vi "Starter Kit 2.0 Roaming - Kinect.vi"() -> ()   [LabVIEW 2010]
doc: "This VI demonstrates how to control the Robotics Starter Kit 2.0 robot. It is deployed to an sbRIO-9632, then run on the Real-Time controller."
uses:
  <vilib>/Utility/AngleManip/NI_AngleManipulation.lvlib
  <vilib>/Utility/AngleManip/Degrees to Radians (Scalar DBL).vi
  <vilib>/Platform/TimedLoop/XDataNode/XDataNode.xnode
  <vilib>/Platform/TimedLoop/XDataNode/timing_clust.ctl
  <vilib>/Platform/TimedLoop/XDataNode/XDNodeRunTimeDep.lvlib
  <vilib>/Platform/TimedLoop/XDataNode/wakeup.ctl
  <vilib>/Platform/TimedLoop/XDataNode/nitl_modes.ctl
  <vilib>/robotics/Steering/Steering Frame/NI_Robotics_Steering Frame.lvclass
  <vilib>/robotics/Steering/Steering Frame/Apply Steering Frame Velocity to Motors.vi
  <vilib>/robotics/Starter Kit/Host Interface/NI_Robotics_Starter Kit Host.lvclass
  <vilib>/robotics/Utilities/Scan Angles/NI_Robotics_Scan Angles.lvlib
  <vilib>/robotics/Starter Kit/2.0/NI_Robotics_Starter Kit Host_2.0.lvlib
  <vilib>/robotics/Starter Kit/2.0/9632 Host Interface/NI_Robotics_Starter Kit Host_9632_2.0.lvclass
  <vilib>/robotics/Obstacle Avoidance/Simple Vector Field Histogram/Gap Description.ctl
  <vilib>/robotics/Obstacle Avoidance/Simple Vector Field Histogram/NI_Robotics_Simple Vector Field Histogram.lvlib
  <vilib>/robotics/Obstacle Avoidance/Simple Vector Field Histogram/Obstacle Description.ctl
  Kinect VIs/Kinect Heading Data.ctl
panel:
  out "Sensor Data":cluster{"angles (deg)":dbl[], "distances":dbl[]}(graph)
  in  "stop":bool
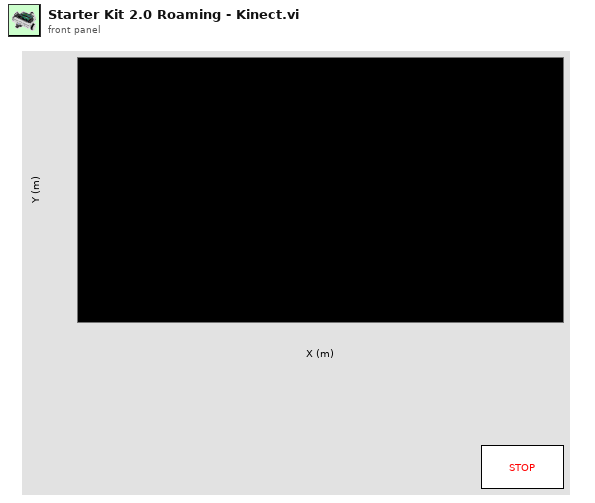
[diagram p1: front panel]
types:
  T1 = typedef "Kinect Heading Data.ctl" = cluster{"largest gap":T2, "nearest obstacle":T3, "obstacle within panic range":bool}
  T2 = typedef "NI_Robotics_Simple Vector Field Histogram.lvlib/Gap Description.ctl" = cluster{"angle to gap":dbl, "size of gap":dbl}
  T3 = typedef "NI_Robotics_Simple Vector Field Histogram.lvlib/Obstacle Description.ctl" = cluster{"angle to obstacle":dbl, "distance to obstacle":dbl}
  T4 = typedef "XDNodeRunTimeDep.lvlib/timing_clust.ctl" = cluster{"Expected End [f-1]":u64, "Actual End [f-1]":u64, "Finished Late? [f-1]":bool, "Expected End [i-1]":u64, "Actual End [i-1]":u64, "Finished Late? [i-1]":bool, "Expected Start [i]":u64, "Actual Start [i]":u64, "Expected Start [f]":u64, "Actual Start [f]":u64, "Source Name":string, "Structure Name":string, "Period":i64, "Deadline":i64, "Offset":i64, "Start":i64, "Priority":i32, "Timeout":i32, "Mode":T5, "Wakeup Reason":T6, "Error":errorcluster, "Source Type":string, "Secondary Source Type":string, "Global End Time":u64, "Global Start Time":u64, "Frame Duration":u64, "Iteration Duration":u64, "Assigned CPU":i32, "I/O Scan Engine Mode":u32}
  T5 = typedef "XDNodeRunTimeDep.lvlib/nitl_modes.ctl" = enum32{"No Change", "Process missed periods, maintain original phase", "Discard missed periods, maintain original phase", "Process missed periods, ignore original phase", "Discard missed periods, ignore original phase"}
  T6 = typedef "XDNodeRunTimeDep.lvlib/wakeup.ctl" = enum32{"Normal", "Aborted", "Asynchronous wakeup", "Timing source error", "Timed loop error", "Timeout"}
  T7 = typedef "NI_Robotics_Scan Angles.lvlib/Scan Angle Data.ctl" = cluster{"angles":dbl[], "distances":dbl[], "current index":i32, "previous index":i32}
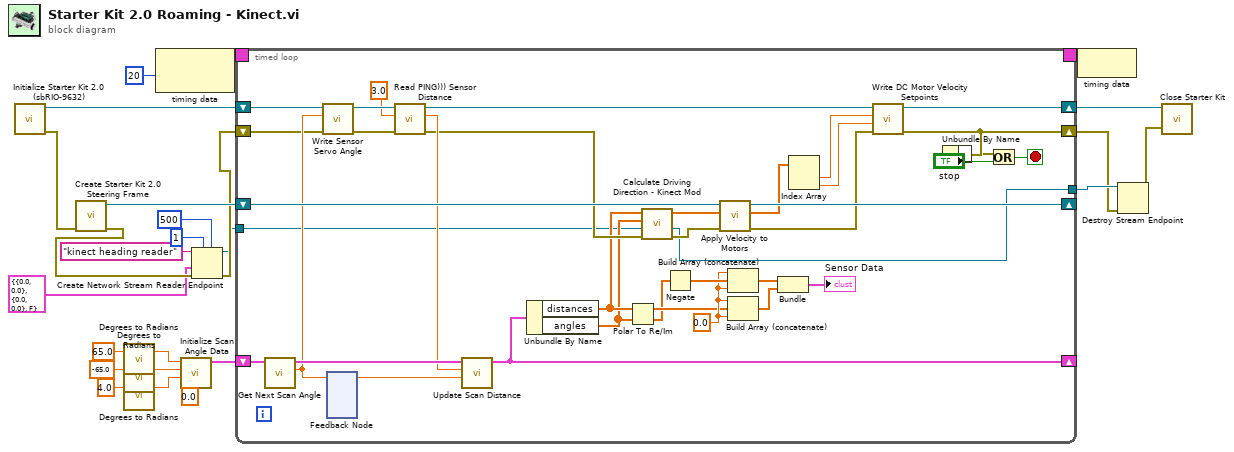
[diagram p0: block diagram]
diagram:
  n1 = call <vilib>:"Initialize Starter Kit 2.0 (sbRIO-9632).vi"() -> ("error out"=w11:errorcluster, "FPGA starter kit host 2.0 out"=w12:refnum<class "NI_Robotics_Starter Kit Host_9632_2.0.lvclass">)  [unwired: 10 in]
  n2 = call <vilib>:"Create Starter Kit 2.0 Steering Frame.vi"("error in (no error)"=w11) -> ("error out"=w7:errorcluster, "starter kit differential steering frame"=w14:refnum<class "NI_Robotics_Differential Steering Frame.lvclass">)  [unwired: 9 in]
  n3 = call-poly <vilib>:"Degrees to Radians.vi"("angle (deg)"=65.0 ("max angle")) -> ("angle (rad)"=w20:dbl)  [unwired: 2 in]
  n4 = call-poly <vilib>:"Degrees to Radians.vi"("angle (deg)"=-65.0 ("min angle")) -> ("angle (rad)"=w16:dbl)  [unwired: 2 in]
  n5 = call-poly <vilib>:"Degrees to Radians.vi"("angle (deg)"=4.0 ("scan angle")) -> ("angle (rad)"=w17:dbl)  [unwired: 2 in]
  n6 = node-c288(i64 20 ("Period")) -> (w25:T4)
  n7 = call <vilib>:"Initialize Scan Angle Data.vi"("initial angle (0)"=0.0, "scan angle"=w17, "min angle"=w16, "max angle"=w20) -> ("scan angles"=w22:T7)  [unwired: 6 in, 1 out]
  n8 = Create Network Stream Reader Endpoint(5:500 ("timeout in ms (-1)"), 7:1 ("reader buffer size"), 8:w7, 9:T1 {"largest gap"={"angle to gap"=0.0, "size of gap"=0.0}, "nearest obstacle"={"angle to obstacle"=0.0, "distance to obstacle"=0.0}, "obstacle within panic range"=FALSE} ("Kinect heading data"), 11:"kinect heading reader" ("reader name")) -> (0:w6:errorcluster, 3:w4:refnum<k21>)  [unwired: 1 in]
  n9 = timed-loop {
    shift-right: [w58] -> _
    shift-left: w22 -> [w60]
    timing: w25 -> [_]
    timing-out: [_] -> w24
    shift-right: [w29] -> w2
    shift-left: w6 -> [w49]
    shift-right: [w46] -> w13
    shift-left: w12 -> [w48]
    shift-right: [w54] -> _
    shift-left: w14 -> [w56]
    tunnel: w4 -> [w28]
    tunnel: [w27] -> w3
    stop <- w62 stop-if-true
    w41 = 0.0 ("element")
    n10 = call <vilib>:"Get Next Scan Angle.vi"("scan angles in"=w60) -> ("new angle"=w52:dbl, "scan angles out"=w59:T7)  [unwired: 9 in]
    n11 = call <vilib>:"Write Sensor Servo Angle.vi"("error in (no error)"=w49, "ccw servo angle (rad)"=w52, "starter kit host in"=w48) -> ("error out"=w31:errorcluster, "starter kit host out"=w32:refnum<class "NI_Robotics_Starter Kit Host_9632_2.0.lvclass">)  [unwired: 7 in]
    n12 = feedback-in #1(w52) -> ()
    n13 = feedback #1() -> (w57:dbl)  [unwired: 1 in]
    n14 = call <vilib>:"Read PING))) Sensor Distance.vi"("error in (no error)"=w31, "default distance (NaN)"=3.0, "starter kit host in"=w32) -> ("error out"=w50:errorcluster, "distance (m)"=w51:dbl, "starter kit host out"=w47:refnum<class "NI_Robotics_Starter Kit Host_9632_2.0.lvclass">)  [unwired: 5 in, 1 out]
    n15 = call <vilib>:"Update Scan Distance.vi"("scan angle"=w57, "new scan distance"=w51, "scan angles in"=w59) -> ("scan angles out"=w58:T7)  [unwired: 8 in]
    n16 = Unbundle By Name(w58) -> ("distances"=w45:dbl[], "angles"=w44:dbl[])
    n17 = Polar To Re/Im(2:w44, 3:w45) -> (0:w38:dbl[], 1:w39:dbl[])
    n18 = call "Calculate Driving Direction - Kinect Mod.vi"("error in (no error)"=w50, "reader endpoint"=w28, "obstacle angles (rad)"=w44, "obstacle distances (m)"=w45) -> ("error out"=w53:errorcluster, "Reader endpoint out"=w27:refnum<k21>, "steering frame velocity"=w55:dbl[])  [unwired: 5 in]
    n19 = Negate(x=w38) -> (-x=w43:dbl[])
    n20 = call-poly <vilib>:"Apply Velocity to Motors.vi"("error in (no error)"=w53, "steering frame velocity"=w55, "steering frame in"=w56) -> ("error out"=w35:errorcluster, "ccw motor velocity setpoints"=w36:dbl[], "steering frame out"=w54:refnum<class "NI_Robotics_Differential Steering Frame.lvclass">)  [unwired: 4 in, 2 out]
    n21 = Build Array (concatenate)(w41, w43, w41) -> (w42:dbl[])
    n22 = Build Array (concatenate)(w41, w39, w41) -> (w40:dbl[])
    n23 = Bundle(w42, w40) -> (→"Sensor Data":cluster{dbl[], dbl[]})  [unwired: 1 in]
    n24 = Index Array(array=w36) -> (element #1=w34:dbl, element #2=w33:dbl)  [unwired: 2 in]
    n25 = call <vilib>:"Write DC Motor Velocity Setpoints.vi"("error in (no error)"=w35, "right motor ccw velocity (rad/s)"=w33, "left motor ccw velocity (rad/s)"=w34, "starter kit host in"=w47) -> ("error out"=w29:errorcluster, "starter kit host out"=w46:refnum<class "NI_Robotics_Starter Kit Host_9632_2.0.lvclass">)  [unwired: 6 in]
    n26 = Or(y="stop") -> (x=w26:errorcluster, x .or. y?=w62:bool)
    n27 = Unbundle By Name(w29, w26) -> ()
  }
  n28 = node-c288(w24) -> ()
  n29 = Destroy Stream Endpoint(8:w2, 11:w3) -> (0:w1:errorcluster)
  n30 = call-dynamic "Close Starter Kit.vi"("error in (no error)"=w1, "starter kit host in"=w13) -> ()  [unwired: 9 in, 1 out]
